vi "QImaging.vi"() -> ()   [LabVIEW 2013]
uses:
  EasyDLL/Debug/EasyDLL.dll
  Debug/QImaging.dll
panel:
  in  "exposure (µs)":u32
  in  "stop":bool
  out "Intensity Graph":u16[][](graph)
  out "paramVal":u32[](array[numeric])
  out "error get info":errorcluster[](array[cluster])
  in  "paramKey IN":u32[](array[numeric])
  out "GetImage error":errorcluster
  out "Config errcode":i32
  out "Config Error":errorcluster
  out "handle":u32
  out "handle close cam":u32
  out "error cam Info":i32
  out "\"closecam\" output":i32
  out "error out close lib":errorcluster
  out "returned ID":u32
  out "error out 4":errorcluster
  out "error out open cam":errorcluster
  out "error out get cams":errorcluster
  out "size of QCam_handle":i32
  out "Camera Id":u32
  out "Number of cameras":string
  out "error out open lib":errorcluster
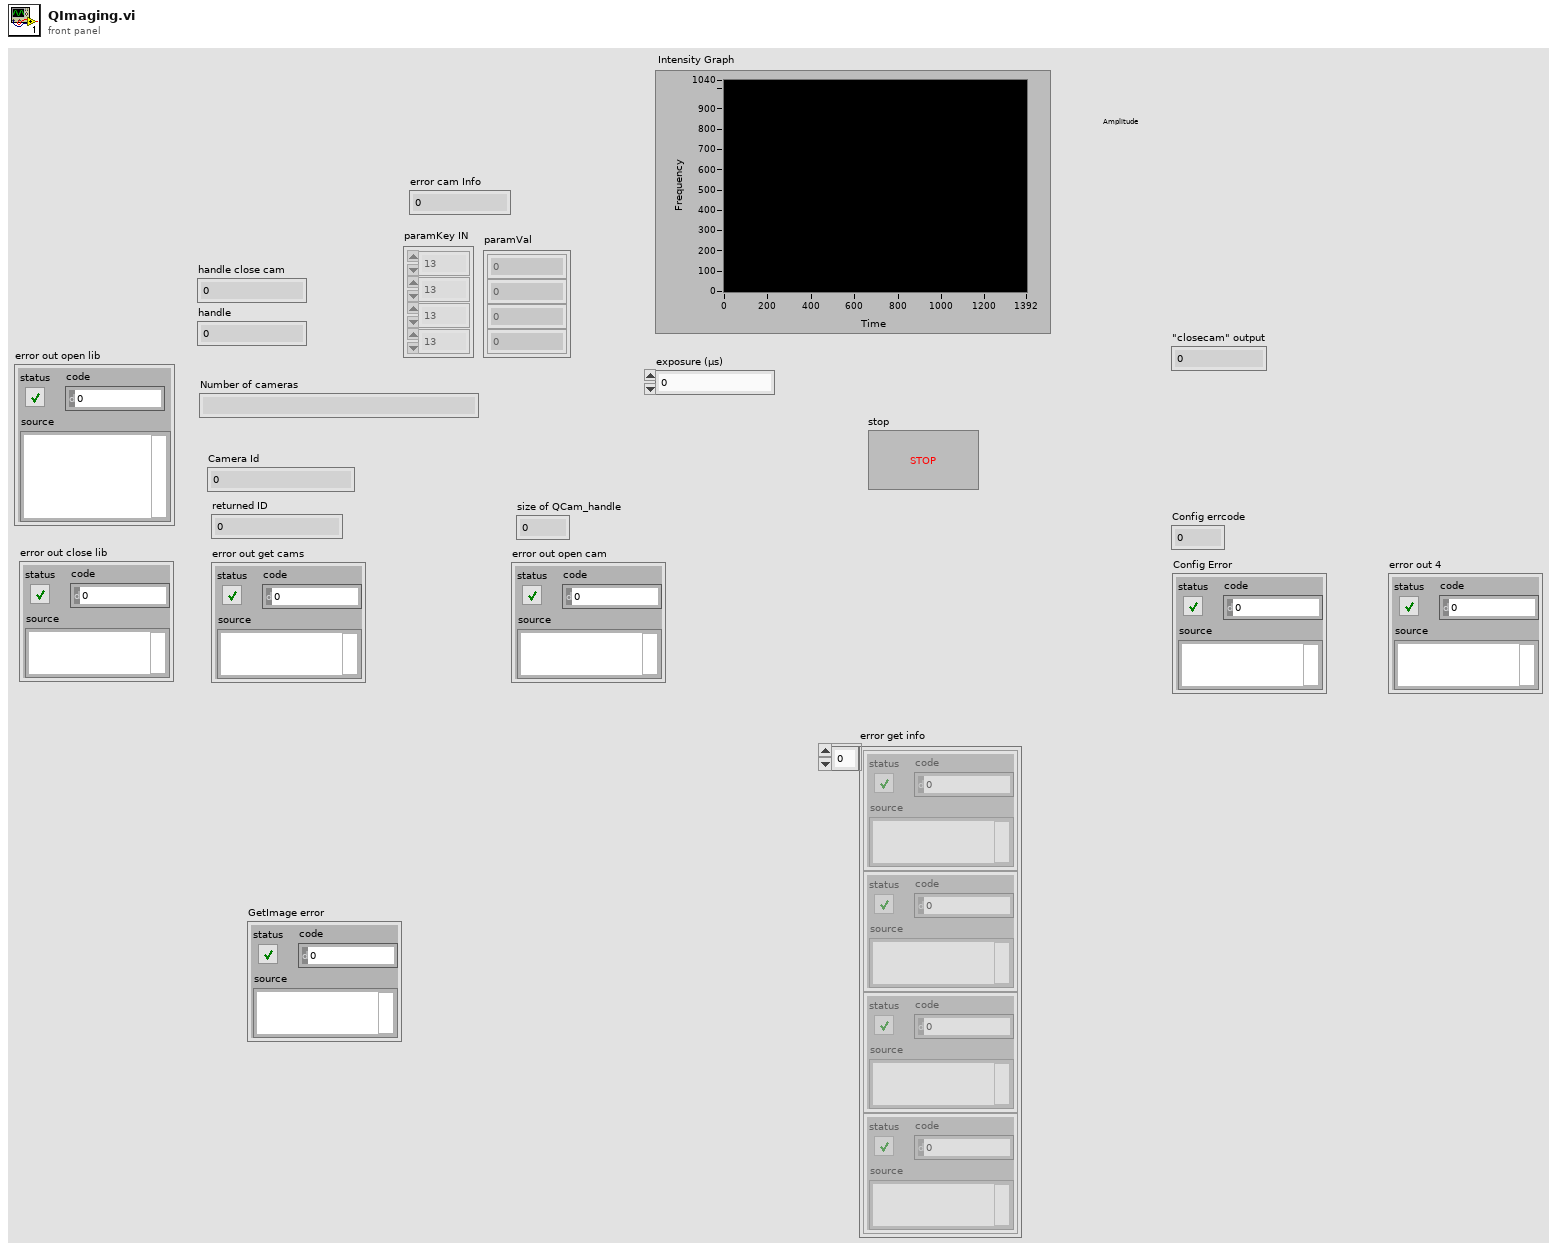
[diagram p1: front panel]
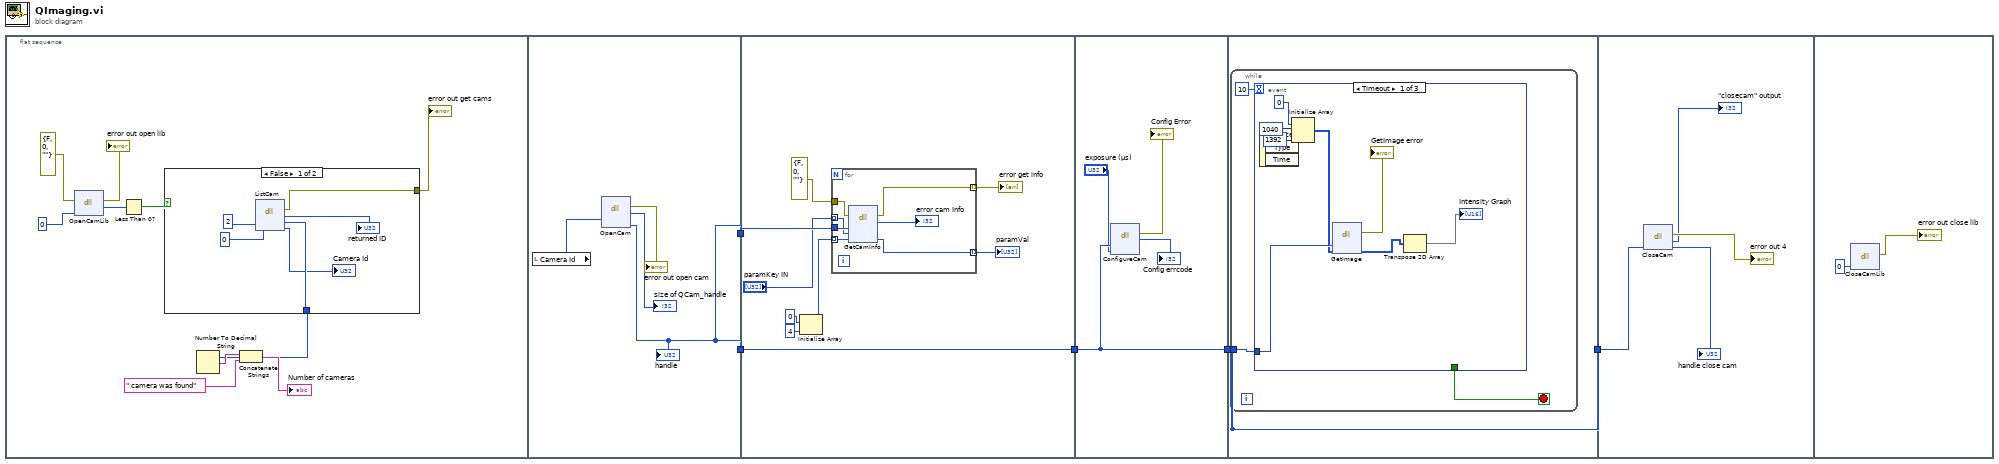
[diagram p0: block diagram]
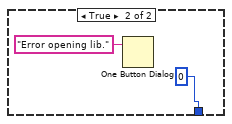
[diagram p2: hidden frame]
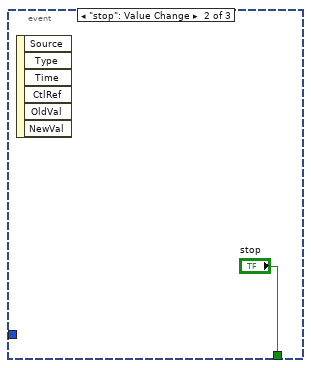
[diagram p3: hidden frame]
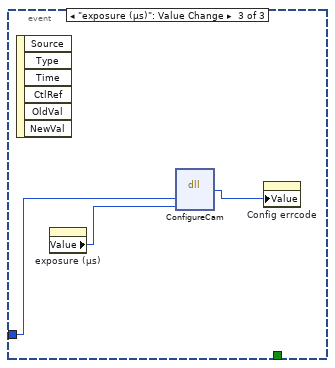
[diagram p4: hidden frame]
diagram:
  n1 = flat-sequence {
    tunnel: [w24] -> w5
    tunnel: [w24] -> w4
    tunnel: w5 -> [w36]
    tunnel: [w36] -> w3
    tunnel: w4 -> [w35]
    tunnel: w3 -> [w47]
    tunnel: [w47] -> w2
    tunnel: w2 -> [w48]
    tunnel: [w48] -> w1
    tunnel: w1 -> [w65]
    frame #0 {
      n2 = dll-call lib="C:/Users/vernier/Documents/Visual Studio 2012/Projects/QImaging/Debug/QImaging.dll" fn="OpenCamLib"(error in=errorcluster {"status"=FALSE, "code"=0, "source"=""} ("error in (no error)"), "i"=0) -> (error out=→"error out open lib":errorcluster, "return type"=w15:i32)  [unwired: 3 in, 1 out]
      n3 = Less Than 0?(x=w15) -> (x < 0?=w14:bool)
      n4 = case shown="False" w14 {
        tunnel: [w21 _] -> w7
        tunnel: [w19 0] -> w8
        frame False {
          n5 = dll-call lib="C:/Users/vernier/Documents/Visual Studio 2012/Projects/QImaging/Debug/QImaging.dll" fn="ListCam"("listLength"=u32 2 ("NumCam"), "cameraId"=u32 0) -> (error out=w21:errorcluster, "return type"=→"returned ID":u32, "listLength"=w19:u32, "cameraId"=→"Camera Id":u32)  [unwired: 3 in, 1 out]
        }
        frame True {
          n6 = One Button Dialog(message="Error opening lib.") -> ()  [unwired: 1 in, 1 out]
        }
      }
      "error out get cams" <- w7
      n7 = Number To Decimal String(number=w8) -> (decimal integer string=w11:string)  [unwired: 1 in]
      n8 = Concatenate Strings(w11, " camera was found" ("message")) -> (→"Number of cameras":string)
    }
    frame #1 {
      n9 = local read "Camera Id"() -> (w25:u32)
      n10 = dll-call lib="C:/Users/vernier/Documents/Visual Studio 2012/Projects/QImaging/Debug/QImaging.dll" fn="OpenCam"("cameraid"=w25) -> (error out=→"error out open cam":errorcluster, "return type"=→"size of QCam_handle":i32, "handle"=w24:u32)  [unwired: 5 in, 1 out]
      "handle" <- w24
    }
    frame #2 {
      n11 = Initialize Array(u32 0, 4 ("dimension size")) -> (w32:u32[])
      n12 = for {
        tunnel: w35 -> [w43]
        tunnel: w32 -> [w41] mode=indexing
        tunnel: "paramKey IN" -> [w40] mode=indexing
        tunnel: errorcluster {"status"=FALSE, "code"=0, "source"=""} ("error out") -> [w39]
        tunnel: [w38] -> w29 mode=indexing
        tunnel: [w37] -> w28 mode=indexing
        n13 = dll-call lib="C:/Users/vernier/Documents/Visual Studio 2012/Projects/QImaging/Debug/QImaging.dll" fn="GetCamInfo"(error in=w39, "handle"=w43, "paramKey"=w40, "paramVal"=w41) -> (error out=w38:errorcluster, "return type"=→"error cam Info":i32, "paramVal"=w37:u32)  [unwired: 4 in, 1 out]
      }
      "error get info" <- w29
      "paramVal" <- w28
    }
    frame #3 {
      n14 = dll-call lib="C:/Users/vernier/Documents/Visual Studio 2012/Projects/QImaging/Debug/QImaging.dll" fn="ConfigureCam"("handle"=w47, "exposure time"="exposure (µs)") -> (error out=→"Config Error":errorcluster, "return type"=→"Config errcode":i32)  [unwired: 5 in, 1 out]
    }
    frame #4 {
      n15 = while {
        tunnel: w48 -> [w51]
        stop <- w50 stop-if-true
        n16 = event shown="[0] Timeout" {
          selector: _ -> [_ _ _]
          dyn-events: _ -> [_ _ _]
          timeout: 10 -> [_ _ _]
          tunnel: w51 -> [w59 _ w63]
          tunnel: [_ "stop" _] -> w50
          event Timeout {
            n17 = event-data() -> ()  [unwired: 1 in, 3 out]
            n18 = Initialize Array(u16 0 ("element"), 1040 ("dimension size"), 1392 ("dimension size")) -> (w54:u16[][])
            n19 = dll-call lib="C:/Users/vernier/Documents/Visual Studio 2012/Projects/QImaging/Debug/QImaging.dll" fn="GetImage"("handle"=w59, "data"=w54) -> (error out=→"GetImage error":errorcluster, "data"=w53:u16[][])  [unwired: 5 in, 1 out]
            n20 = Transpose 2D Array(2D array=w53) -> (transposed array=→"Intensity Graph":u16[][])
          }
          event "stop": Value Change {
            n21 = event-data() -> ()  [unwired: 1 in, 6 out]
          }
          event "exposure (µs)": Value Change {
            n22 = event-data() -> ()  [unwired: 1 in, 6 out]
            n23 = property on="exposure (µs)" class="DigNum (strict)"() -> ("Value"=w62:u32)  [unwired: 2 in, 2 out]
            n24 = dll-call lib="C:/Users/vernier/Documents/Visual Studio 2012/Projects/EasyDLL/Debug/EasyDLL.dll" fn="ConfigureCam"("handle"=w63, "exposure time"=w62) -> ("return type"=w61:i32)  [unwired: 5 in, 2 out]
            n25 = property on="Config errcode" class="DigNum (strict)"("Value"=w61) -> ()  [unwired: 2 in, 2 out]
          }
        }
      }
    }
    frame #5 {
      n26 = dll-call lib="C:/Users/vernier/Documents/Visual Studio 2012/Projects/QImaging/Debug/QImaging.dll" fn="CloseCam"("handle"=w65) -> (error out=→"error out 4":errorcluster, "return type"=→"\"closecam\" output":i32, "handle"=→"handle close cam":u32)  [unwired: 3 in, 1 out]
    }
    frame #6 {
      n27 = dll-call lib="C:/Users/vernier/Documents/Visual Studio 2012/Projects/QImaging/Debug/QImaging.dll" fn="CloseCamLib"("i"=0) -> (error out=→"error out close lib":errorcluster)  [unwired: 5 in, 1 out]
    }
  }
